vi "Renishaw-XL80_SetUpdateAirCompMethod.vi"(8 "error in (no error)":errorcluster, 11 "Renishaw-XL80 in":refnum<class "Renishaw-XL80.lvclass">) -> (0 "error out":errorcluster, 3 "Renishaw-XL80 out":refnum<class "Renishaw-XL80.lvclass">)   [LabVIEW 2024, in "Renishaw-XL80.lvclass"]
doc: "This method updates the material compensation factor using the most recently acquired material temperature sensor readings.\n\nDefinition\nHRESULTUpdateMatComp();\nParameters\nNone\n\nComments\nThis method will return with an HRESULT of E_FAIL if AutoCompensationMode is set to AUTO_COMPENSATION_FULL. This warns the client that calculating the material compensation factor whilst it is being automatically updated is somewhat pointless.\n\nThis method will also return E_FAIL if the EC10 is disconnected.\n\nIf successful this method will return an HRESULT of S_OK."
uses:
  Renishaw-XL80.lvclass
  Renishaw-XL80.lvclass/Renishaw-XL80.ctl
  D:/A.C.M/Example CSharp_64/bin/Debug/Interop.DX10SDKADAPTORLib.dll
  Example CSharp_64/bin/Debug/Interop.DX10SDKADAPTORLib.dll
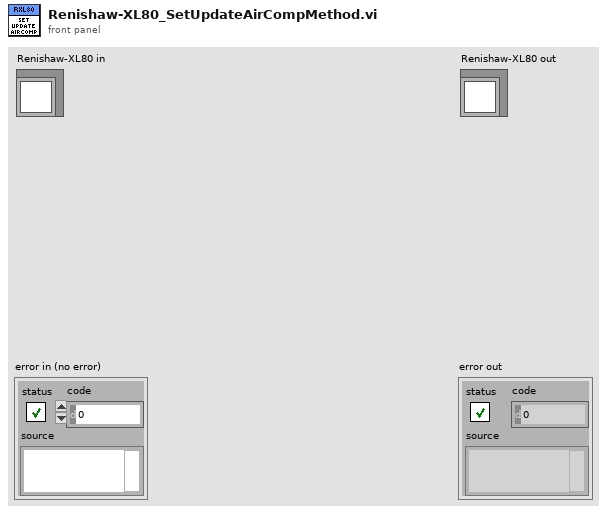
[diagram p1: front panel]
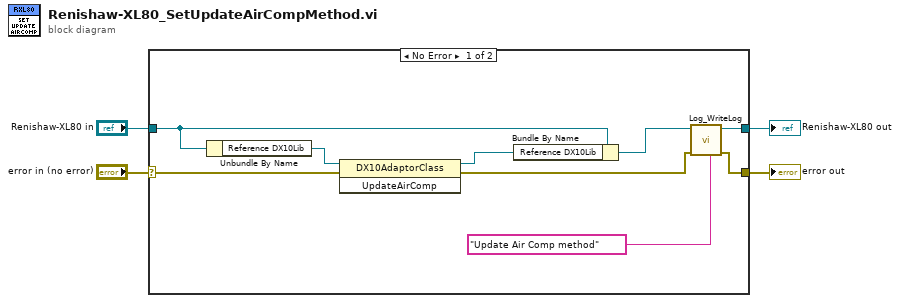
[diagram p0: block diagram]
diagram:
  n1 = case shown="No Error" "error in (no error)" {
    selector: "error in (no error)" -> [w8 w15]
    tunnel: [w6 w15] -> w3
    tunnel: [w7 w14] -> w1
    tunnel: "Renishaw-XL80 in" -> [w5 w14]
    frame No Error {
      n2 = Unbundle By Name(w5) -> ("Reference DX10Lib"=w13:refnum<k24>)
      n3 = invoke class="DX10AdaptorClass" method="UpdateAirComp"(reference=w13, error in=w8) -> (reference out=w11:refnum<k24>, error out=w10:errorcluster)  [unwired: 1 in, 1 out]
      n4 = Bundle By Name(cluster=w5, "Reference DX10Lib"=w11) -> (w12:refnum<class "Renishaw-XL80.lvclass">)
      n5 = call-dynamic "Log_WriteLog.vi"("Additional text"="Update Air Comp method", "error in (no error)"=w10, "Log in"=w12) -> ("error out"=w6:errorcluster, "Log out"=w7:refnum<class "Renishaw-XL80.lvclass">)  [unwired: 7 in]
    }
    frame Error {
    }
  }
  "error out" <- w3
  "Renishaw-XL80 out" <- w1
